vi "Waveform Buffer Generation.vi"(4 "offset":dbl=2.0 caption="Offset" format="%0.2p", 5 "Amplitude":dbl=2.0 format="%0.2p", 6 "Cycles per Buffer":dbl=1.0 format="%.2f", 7 "Samples per Buffer":dbl=1000.0, 8 "error in (no error)":errorcluster, 9 "Waveform Type":T1(ring), 10 "Desired Frequency":dbl=1000.0 format="%.2f", 11 "task/channels in":refnum<k21>) -> (0 "error out":errorcluster, 1 "Resulting Frequency":dbl format="%.2f", 2 "Waveform":waveform(dbl)[](array[waveform]), 3 "task out":refnum<k21>)   [LabVIEW 2011]
doc: "This subVI is used to create a Sine, Square, Triangle or Sawtooth Waveform. The inputs to this VI are the Waveform Type, which determines if the output waveform is a Sine, Square, Triangle, or Sawtooth Waveform, the amplitude, Desired Frequency, Samples per Buffer, and Cycles per Buffer. \n\nThe Desired Frequency, Samples per Buffer, and Cycles per Buffer are used to calculate the sample clock rate. The DAQmx Timing property node sets the sample clock rate for the device specified in the task/channels in control. \n\nThe actual, coerced, sample clock rate is returned and used as an input to the Basic Function Generator.vi. The Basic Function Generator returns a waveform of data with timing information.\n\nThe formula below was used to determine the sample clock rate:\n\nDesired Frequency=[(Cycles/Buffer)X(Sample Clock Rate)]/Samples per Buffer\n\nNote: The Block Diagram rearranges the variables to solve for Sample Clock Rate"
uses:
  <vilib>/measure/NI_MABase.lvlib
  C:/Program Files/National Instruments/LabVIEW 2011/resource/objmgr/daqmx.rc
panel:
  in  "phase":dbl=1.0 caption="Phase" format="%.2f"
  out "Samples/cycle":dbl format="%0.2f"
  out "Desired Sample Clock Rate":dbl format="%.2f"
  out "Resulting Sample Clock Rate":dbl format="%.2f"
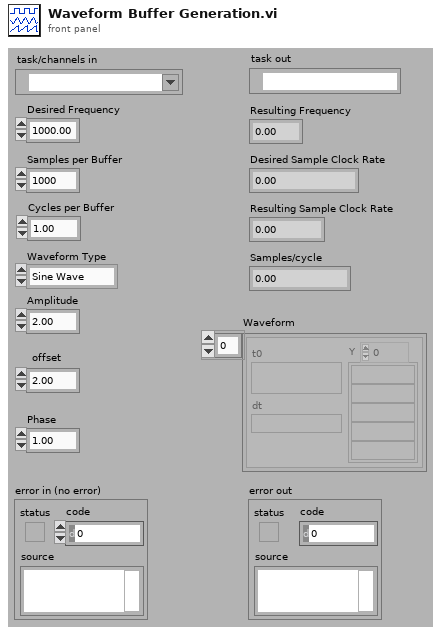
[diagram p1: front panel]
types:
  T1 = enum16{"Sine Wave", "Triangle Wave", "Square Wave", "Sawtooth Wave"}
  T2 = cluster{"SampClk.Rate":dbl, "Samples per Buffer":dbl}
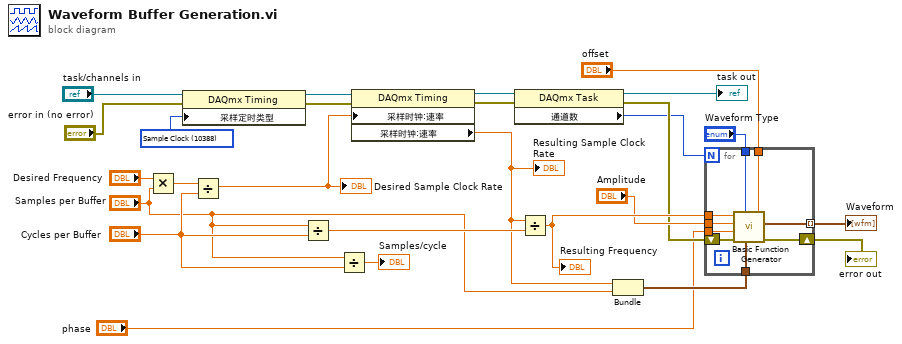
[diagram p0: block diagram]
diagram:
  w12 = 10388 items=["Sample Clock"=10388, "Handshake"=10389, "Implicit"=10451, "On Demand"=10390, "Change Detection"=12504] ("SampTimingType")
  n1 = Multiply(x="Desired Frequency", y="Samples per Buffer") -> (x*y=w23:dbl)
  n2 = property class="DAQmx Timing"(reference="task/channels in", error in="error in (no error)", "采样定时类型"=w12) -> (reference out=w14:refnum<k21>, error out=w13:errorcluster)
  n3 = Divide(x=w23, y="Cycles per Buffer") -> (x/y=w19:dbl)
  "Desired Sample Clock Rate" <- w19
  n4 = Divide(x="Samples per Buffer", y="Cycles per Buffer") -> (x/y=w20:dbl)
  n5 = Divide(x="Samples per Buffer", y="Cycles per Buffer") -> (x/y=→"Samples/cycle":dbl)
  n6 = property class="DAQmx Timing"(reference=w14, error in=w13, "采样时钟:速率"=w19) -> (reference out=w8:refnum<k21>, error out=w9:errorcluster, "采样时钟:速率"=w16:dbl)
  "Resulting Sample Clock Rate" <- w16
  n7 = property class="DAQmx Task"(reference=w8, error in=w9) -> (reference out=→"task out":refnum<k21>, error out=w7:errorcluster, "通道数"=w3:u32)
  n8 = Divide(x=w16, y=w20) -> (x/y=w26:dbl)
  "Resulting Frequency" <- w26
  n9 = Bundle("SampClk.Rate"=w16, "Samples per Buffer"="Samples per Buffer") -> (w24:T2)  [unwired: 1 in]
  n10 = for {
    N: w3 -> [_]
    tunnel: w26 -> [w35]
    tunnel: w24 -> [w34]
    tunnel: [w33] -> w5 mode=indexing
    tunnel: "Amplitude" -> [w32]
    shift-right: [w31] -> w15
    shift-left: w7 -> [w30]
    tunnel: "Waveform Type" -> [w29]
    tunnel: "offset" -> [w28]
    tunnel: "phase" -> [w27]
    n11 = call <vilib>:"Basic Function Generator.vi"("offset"=w28, "sampling info"=w34, "signal type"=w29, "error in (no error)"=w30, "phase"=w27, "amplitude"=w32, "frequency"=w35) -> ("error out"=w31:errorcluster, "signal out"=w33:waveform(dbl))  [unwired: 2 in, 1 out]
  }
  "error out" <- w15
  "Waveform" <- w5
